vi "Configure Test Runner.vi"(8 "error in (no error)":errorcluster, 10 "Number of Test Runners":u32=1, 11 "Execution API In":refnum<class "Execution API.lvclass">) -> (0 "error out":errorcluster, 3 "Execution API Out":refnum<class "Execution API.lvclass">)   [LabVIEW 2020, in "Execution API.lvclass"]
doc: "Configure the number of test runners to launch in parallel. The configuration must be made before running the tests."
uses:
  Execution API.lvclass
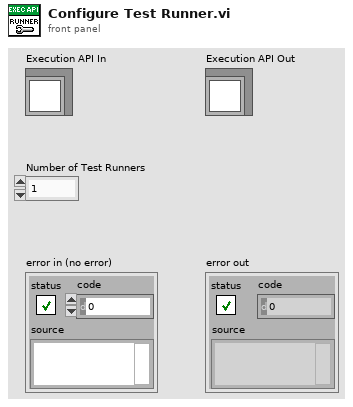
[diagram p1: front panel]
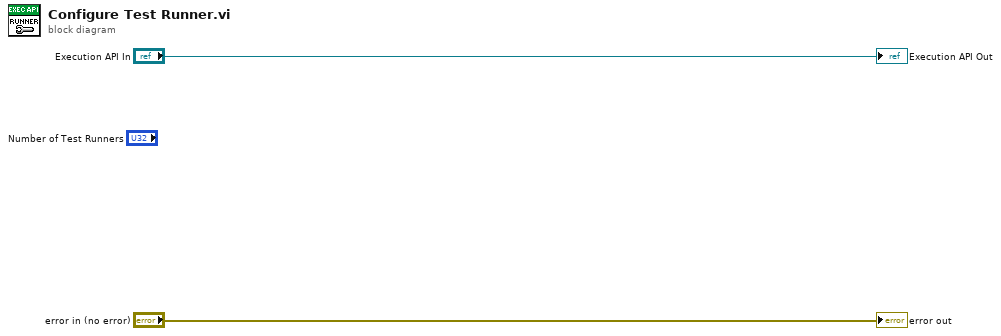
[diagram p0: block diagram]
diagram:
  "error out" <- "error in (no error)"
  "Execution API Out" <- "Execution API In"
